vi "Read Helper Loop DVR.vi"(8 "error in (no error)":errorcluster, 11 "Analog Reader in":refnum<class "Analog Reader.lvclass">) -> (0 "error out":errorcluster, 2 "Helper Loop DVR":refnum<data-value>, 3 "Analog Reader out":refnum<class "Analog Reader.lvclass">)   [LabVIEW 2024]
uses:
  Analog Reader.lvclass/Analog Reader.ctl
  Analog Reader.lvclass
  C:/Users/uspoaotto/OneDrive - Oregon Tool/Desktop/working copies/DAQmxActor/src/DAQmx Actor/DAQmx Actor/DAQmx Actor.lvclass
  C:/Program Files (x86)/National Instruments/LabVIEW 2024/vi.lib/ActorFramework/Actor/Actor.lvclass
  C:/Users/uspoaotto/OneDrive - Oregon Tool/Desktop/working copies/DAQmxActor/src/DAQmx Actor/Analog Reader/Analog Reader.lvclass
  Analog Reader Helper/Analog Reader Helper.lvclass
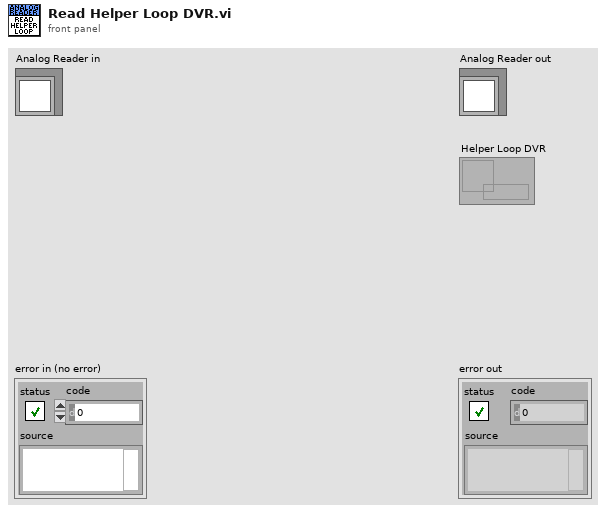
[diagram p1: front panel]
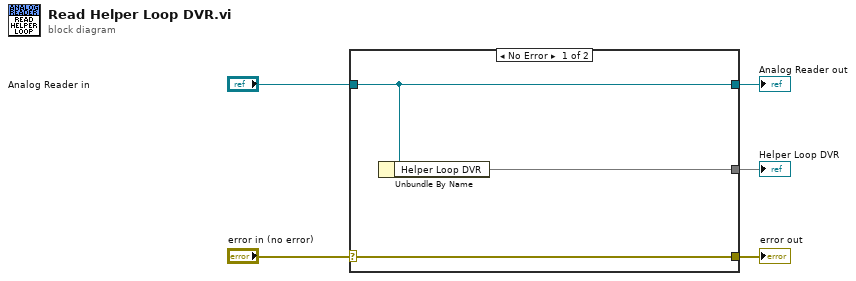
[diagram p0: block diagram]
diagram:
  n1 = case shown="No Error" "error in (no error)" {
    selector: "error in (no error)" -> [w8 w9]
    tunnel: [w8 w9] -> w4
    tunnel: [w7 w10] -> w2
    tunnel: "Analog Reader in" -> [w7 w10]
    tunnel: [w6 _] -> w1
    frame No Error {
      n2 = Unbundle By Name(w7) -> ("Helper Loop DVR"=w6)
    }
    frame Error {
    }
  }
  "error out" <- w4
  "Analog Reader out" <- w2
  "Helper Loop DVR" <- w1
